vi "Test2.vi"() -> ()   [LabVIEW 2024]
uses:
  Automation Controller/Automation Controller/Automation Controller.lvclass
  C:/Program Files (x86)/National Instruments/LabVIEW 2024/vi.lib/ActorFramework/Actor/Actor.lvclass
  <vilib>/ActorFramework/Message Enqueuer/Message Enqueuer.lvclass/Message Enqueuer.ctl
  <vilib>/ActorFramework/Message Enqueuer/Enqueue.vi
  Automation Controller/Automation Controller Messages/Start Cycle Msg/Start Cycle Msg.lvclass
  C:/Program Files (x86)/National Instruments/LabVIEW 2024/vi.lib/ActorFramework/Message/Message.lvclass
  Automation Controller/Automation Controller Messages/Cycle Complete Msg/Cycle Complete Msg.lvclass
  <vilib>/ActorFramework/Stop Msg/Stop Msg.lvclass
  Automation Controller/Automation Controller Messages/Logging Active Msg/Logging Active Msg.lvclass
  Automation Controller/Automation Controller Messages/Logging Stopped Msg/Logging Stopped Msg.lvclass
  <vilib>/ActorFramework/Message Priority Queue/Priority Enqueue.vi
  <vilib>/ActorFramework/Actor/Actor.lvclass
panel:
  in  "Logging Stopped":bool
  in  "Logging Active":bool
  in  "Stop":bool
  in  "Cycle Complete":bool
  in  "Start Cycle":bool
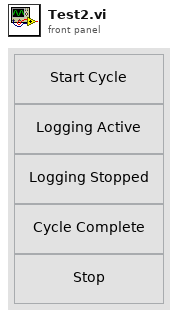
[diagram p1: front panel]
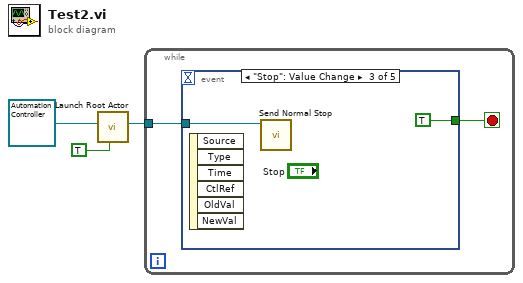
[diagram p0: block diagram]
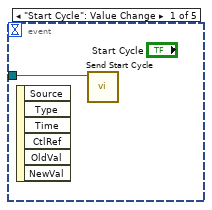
[diagram p2: hidden frame]
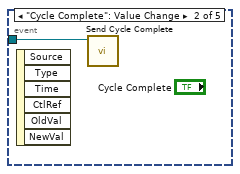
[diagram p3: hidden frame]
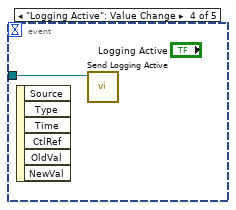
[diagram p4: hidden frame]
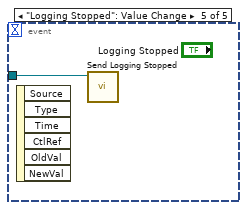
[diagram p5: hidden frame]
diagram:
  n1 = call <vilib>:"Launch Root Actor.vi"("Open Actor Core front panel? (F)"=TRUE, "Actor"=refnum<class "Automation Controller.lvclass"> refnum ("Automation Controller.lvlib:Automation Controller.lvclass")) -> ("Actor's Enqueuer"=w1:refnum<class "Message Enqueuer.lvclass">)  [unwired: 8 in, 1 out]
  n2 = while {
    tunnel: w1 -> [w4]
    stop <- w5 stop-if-true
    n3 = event shown="[2] \"Stop\": Value Change" {
      selector: _ -> [_ _ _ _ _]
      dyn-events: _ -> [_ _ _ _ _]
      timeout: _ -> [_ _ _ _ _]
      tunnel: [_ _ TRUE _ _] -> w5
      tunnel: w4 -> [w6 w7 w8 w10 w11]
      event "Start Cycle": Value Change {
        n4 = event-data() -> ()  [unwired: 1 in, 6 out]
        n5 = call "Send Start Cycle.vi"("Message Enqueuer"=w6) -> ()  [unwired: 9 in, 2 out]
      }
      event "Cycle Complete": Value Change {
        n6 = event-data() -> ()  [unwired: 1 in, 6 out]
        n7 = call "Send Cycle Complete.vi"("Message Enqueuer"=w7) -> ()  [unwired: 9 in, 2 out]
      }
      event "Stop": Value Change {
        n8 = event-data() -> ()  [unwired: 1 in, 6 out]
        n9 = call <vilib>:"Send Normal Stop.vi"("Message Enqueuer"=w8) -> ()  [unwired: 10 in, 1 out]
      }
      event "Logging Active": Value Change {
        n10 = event-data() -> ()  [unwired: 1 in, 6 out]
        n11 = call "Send Logging Active.vi"("Message Enqueuer"=w10) -> ()  [unwired: 9 in, 2 out]
      }
      event "Logging Stopped": Value Change {
        n12 = event-data() -> ()  [unwired: 1 in, 6 out]
        n13 = call "Send Logging Stopped.vi"("Message Enqueuer"=w11) -> ()  [unwired: 9 in, 2 out]
      }
    }
  }
